vi "Pid.vi"() -> ()   [LabVIEW 2016]
uses:
  <vilib>/Instr/_visa.llb/VISA Configure Serial Port (Instr).vi
panel:
  out "String 2":string
  out "String":string
  out "CM4SpeedPID.ref":i16
  out "CM3SpeedPID.ref":i16
  out "CM2SpeedPID.ref":i16
  out "CM1SpeedPID.ref":i16
  out "ChassisData.ChassisSpeedRef.Omega":i16
  out "ChassisData.ChassisSpeedRef.X":i16
  out "ChassisData.ChassisSpeedRef.Y":i16
  out "GMPitchEncoder.ecd_angle":i16
  out "GMYawEncoder.ecd_angle":i16
  out "GMYawEncoder.ecd_bias":i16
  out "GMYawEncoder.raw_value":i16
  out "GMPitchEncoder.ecd_bias":i16
  out "GMPitchEncoder.raw_value":i16
  out "GMPPositionPID.fdb":i16
  out "GMYPositionPID.fdb":i16
  out "GMPSpeedPID.fdb":i16
  out "GMYSpeedPID.fdb":i16
  out "GMPPositionPID.ref":i16
  out "GMYPositionPID.ref":i16
  out "GMPSpeedPID.ref":i16
  out "GMYSpeedPID.ref":i16
  out "Motor4_Measure.speed_rpm":i16
  out "Motor3_Measure.speed_rpm":i16
  out "Motor2_Measure.speed_rpm":i16
  out "Motor1_Measure.speed_rpm":i16
  out "RC_CtrlData.mouse.y":i16
  out "RC_CtrlData.mouse.x":i16
  out "RC_CtrlData.key.v":i16
  out "RC_CtrlData.rc.s2":i16
  out "RC_CtrlData.rc.s1":i16
  out "RC_CtrlData.rc.ch3":i16
  out "RC_CtrlData.rc.ch1":i16
  out "RC_CtrlData.rc.ch0":i16
  out "RC_CtrlData.rc.ch2":i16
  out "MPU6050_Raw_Data.Gyro_Z":i16
  out "AppParamRealUsed.GyroCaliData.GyroZOffset":i16
  out "AppParamRealUsed.GyroCaliData.GyroYOffset":i16
  out "AppParamRealUsed.GyroCaliData.GyroXOffset":i16
  out "MPU6050_Raw_Data.Gyro_Y":i16
  out "MPU6050_Raw_Data.Gyro_X":i16
  out "MPU6050_Raw_Data.Accel_Z":i16
  out "MPU6050_Raw_Data.Accel_Y":i16
  out "MPU6050_Raw_Data.Accel_X":i16
  out "yaw_angle":i16
  out "roll_angle":i16
  out "pitch_angle":i16
  out "GetChassis_MoveMode":u16
  out "GetGimbal_MoveMode":u16
  out "GetShootState":u16
  out "GetFrictionState":u16
  out "GetAttackMode":u16
  out "GetWorkState":u16
  out "Chassis_MoveMode":string="Nothing"
  out "Gimbal_MoveMode":string="Nothing"
  out "ShootState":string="Nothing"
  out "FrictionState":string="Nothing"
  out "AttackMode":string="Nothing"
  out "WorkState":string="Nothing"
  out "DBUSFrameRate":i16
  out "PitchFrameRate":i16
  out "YawFrameRate":i16
  out "ChassisFrameRate[0]":i16
  out "ChassisFrameRate[1]":i16
  out "ChassisFrameRate[2]":i16
  out "ChassisFrameRate[3]":i16
  out "JudgeFrameRate":i16
  out "IMUFrameRate":i16
  out "MiniPCFrameRate":i16
  out "show num":u32
  out "Init":u8
  out "First?":bool=TRUE
  out "Waveform Chart":dynamicdata(graph)
  in  "ID:":u8=2 format="%x"
  in  "Save":bool
  in  "Show":bool
  in  "File Name:":string="Frame"
  in  "Open":bool
  in  "Baud Rate":u32(ring)=115200 items=["76800"=76800, "100000"=100000, "500000"=500000, "115200"=115200, "9600"=9600]
  in  "Serial port":refnum<visa-resource-name>
  out "Wrong":u64
  out "Right":u64
  in  "unpack":T1 {"Data" format="%x"; "Frame length" format="%x"; "Frame ID" format="%x"}
  in  "Tab Control":enum32{"Gimbal", "Shoot", "Chassis"}(tab)
  in  "Down Picth":bool
  in  "Down Yaw":bool
  out "Down Picth Susess":bool caption="Picth susess"
  out "Down Yaw Susess":bool caption="Picth susess"
  out "Y-S-D 3":u16
  out "Y-S-I 3":u16
  out "Y-S-P 3":u16
  out "Y-P-D 3":u16
  out "Y-P-I 3":u16
  out "Y-P-P 3":u16
  out "P-P-P 3":u16
  out "P-S-D 3":u16
  out "P-S-I 3":u16
  out "P-S-P 3":u16
  out "P-P-D 3":u16
  out "P-P-I 3":u16
  in  "P-P-P 2":u16
  in  "Y-S-D 2":u16
  in  "Y-S-I 2":u16
  in  "Y-S-P 2":u16
  in  "Y-P-D 2":u16
  in  "Y-P-I 2":u16
  in  "Y-P-P 2":u16
  in  "P-S-D 2":u16
  in  "P-S-I 2":u16
  in  "P-S-P 2":u16
  in  "P-P-D 2":u16
  in  "P-P-I 2":u16
  in  "S-P-I":u16
  in  "S-P-D":u16
  in  "S-S-P":u16
  in  "S-S-I":u16
  in  "S-S-D":u16
  in  "S-P-P":u16
  out "S-P-I 4":u16
  out "S-P-D 4":u16
  out "S-S-P 4":u16
  out "S-S-I 4":u16
  out "S-S-D 4":u16
  out "S-P-P 4":u16
  out "T-T-T-S 4":u16
  out "F-W-M-V 4":u16
  out "Down Shoot Susess":bool caption="Picth susess"
  in  "Down Shoot":bool
  in  "T-T-T-S":u16
  in  "F-W-M-V":u16
  in  "R-S-I":u16
  in  "R-S-D":u16
  in  "C-S-P":u16
  in  "C-S-I":u16
  in  "C-S-D":u16
  in  "R-S-P":u16
  out "R-S-I 5":u16
  out "R-S-D 5":u16
  out "C-S-P 5":u16
  out "C-S-I 5":u16
  out "C-S-D 5":u16
  out "R-S-P 5":u16
  out "Down Chassis Susess":bool caption="Picth susess"
  in  "Down Chassis":bool
  in  "Calibrate Gimbal":bool
  out "Calibrate Gimbal Susess":bool caption="Picth susess"
  in  "Calibrate Gyro":bool
  out "Calibrate Gyro Susess":bool caption="Picth susess"
  in  "Calibrate LittleGyro":bool
  out "Calibrate LittleGyro Susess":bool caption="Picth susess"
  # "Position"
  # "Speed"
  # "Position"
  # "Speed"
  # "Pitch"
  # "Yaw"
  # "Pitch"
  # "Yaw"
  # "Position"
  # "Speed"
  # "Position"
  # "Speed"
  # "Turn\nTable"
  # "Turn\nTable"
  # "Turn Table\nTarget speed"
  # "Turn Table\nTarget speed"
  # "Friction Wheel\nMax Value"
  # "Friction Wheel\nMax Value"
  # "Position"
  # "Speed"
  # "Position"
  # "Speed"
  # "Chassis"
  # "Chassis"
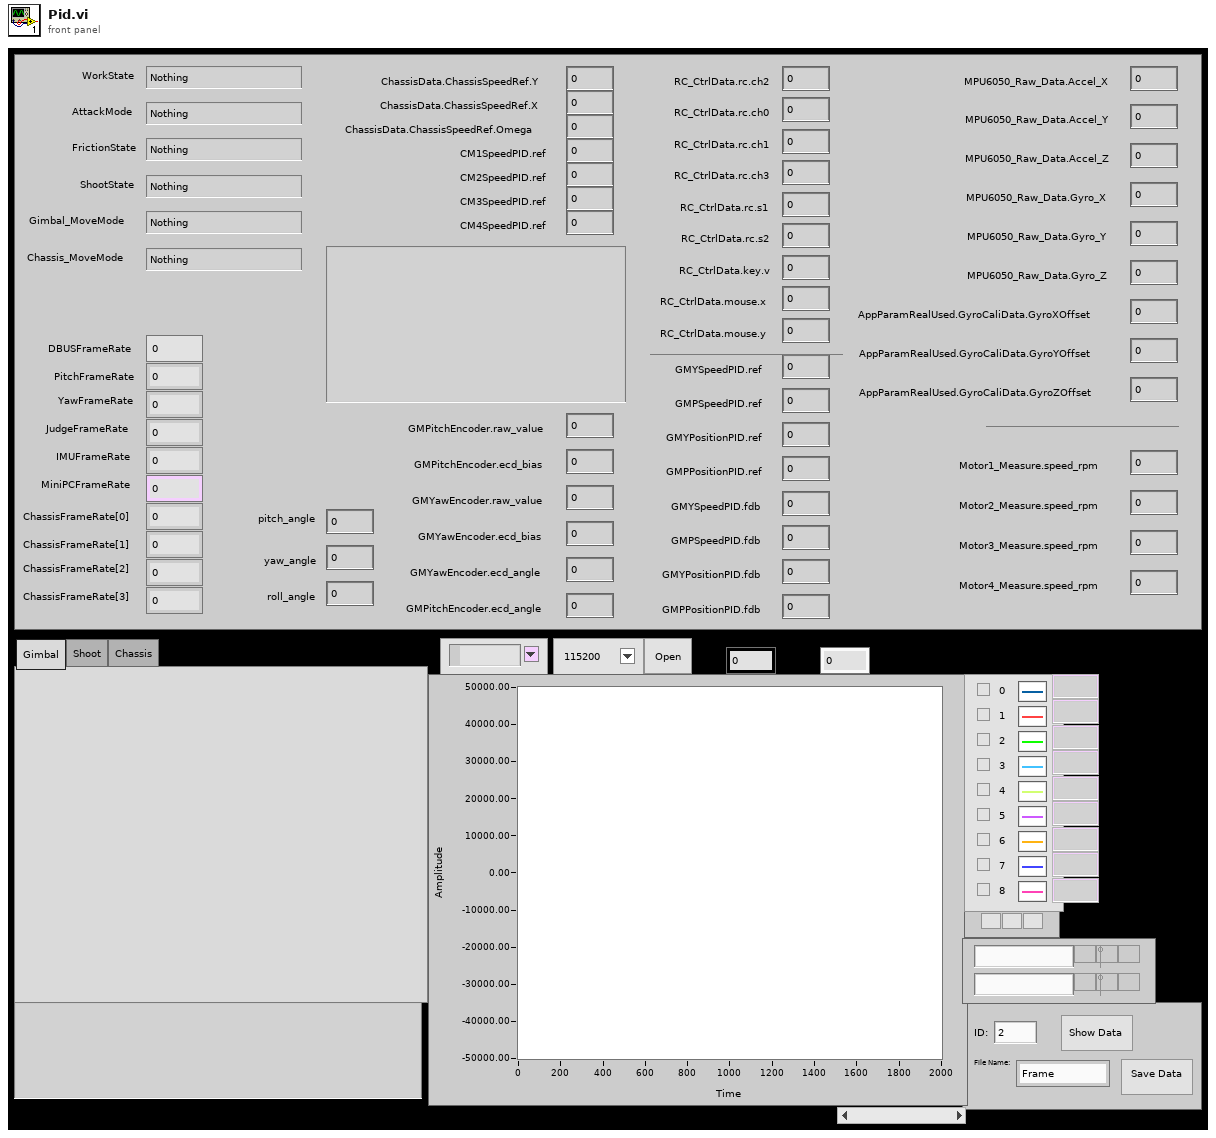
[diagram p1: front panel]
types:
  T1 = cluster{"Status":u8, "Read":u8, "Frame ID":u8, "Frame length":u8, "Data":u8[]}
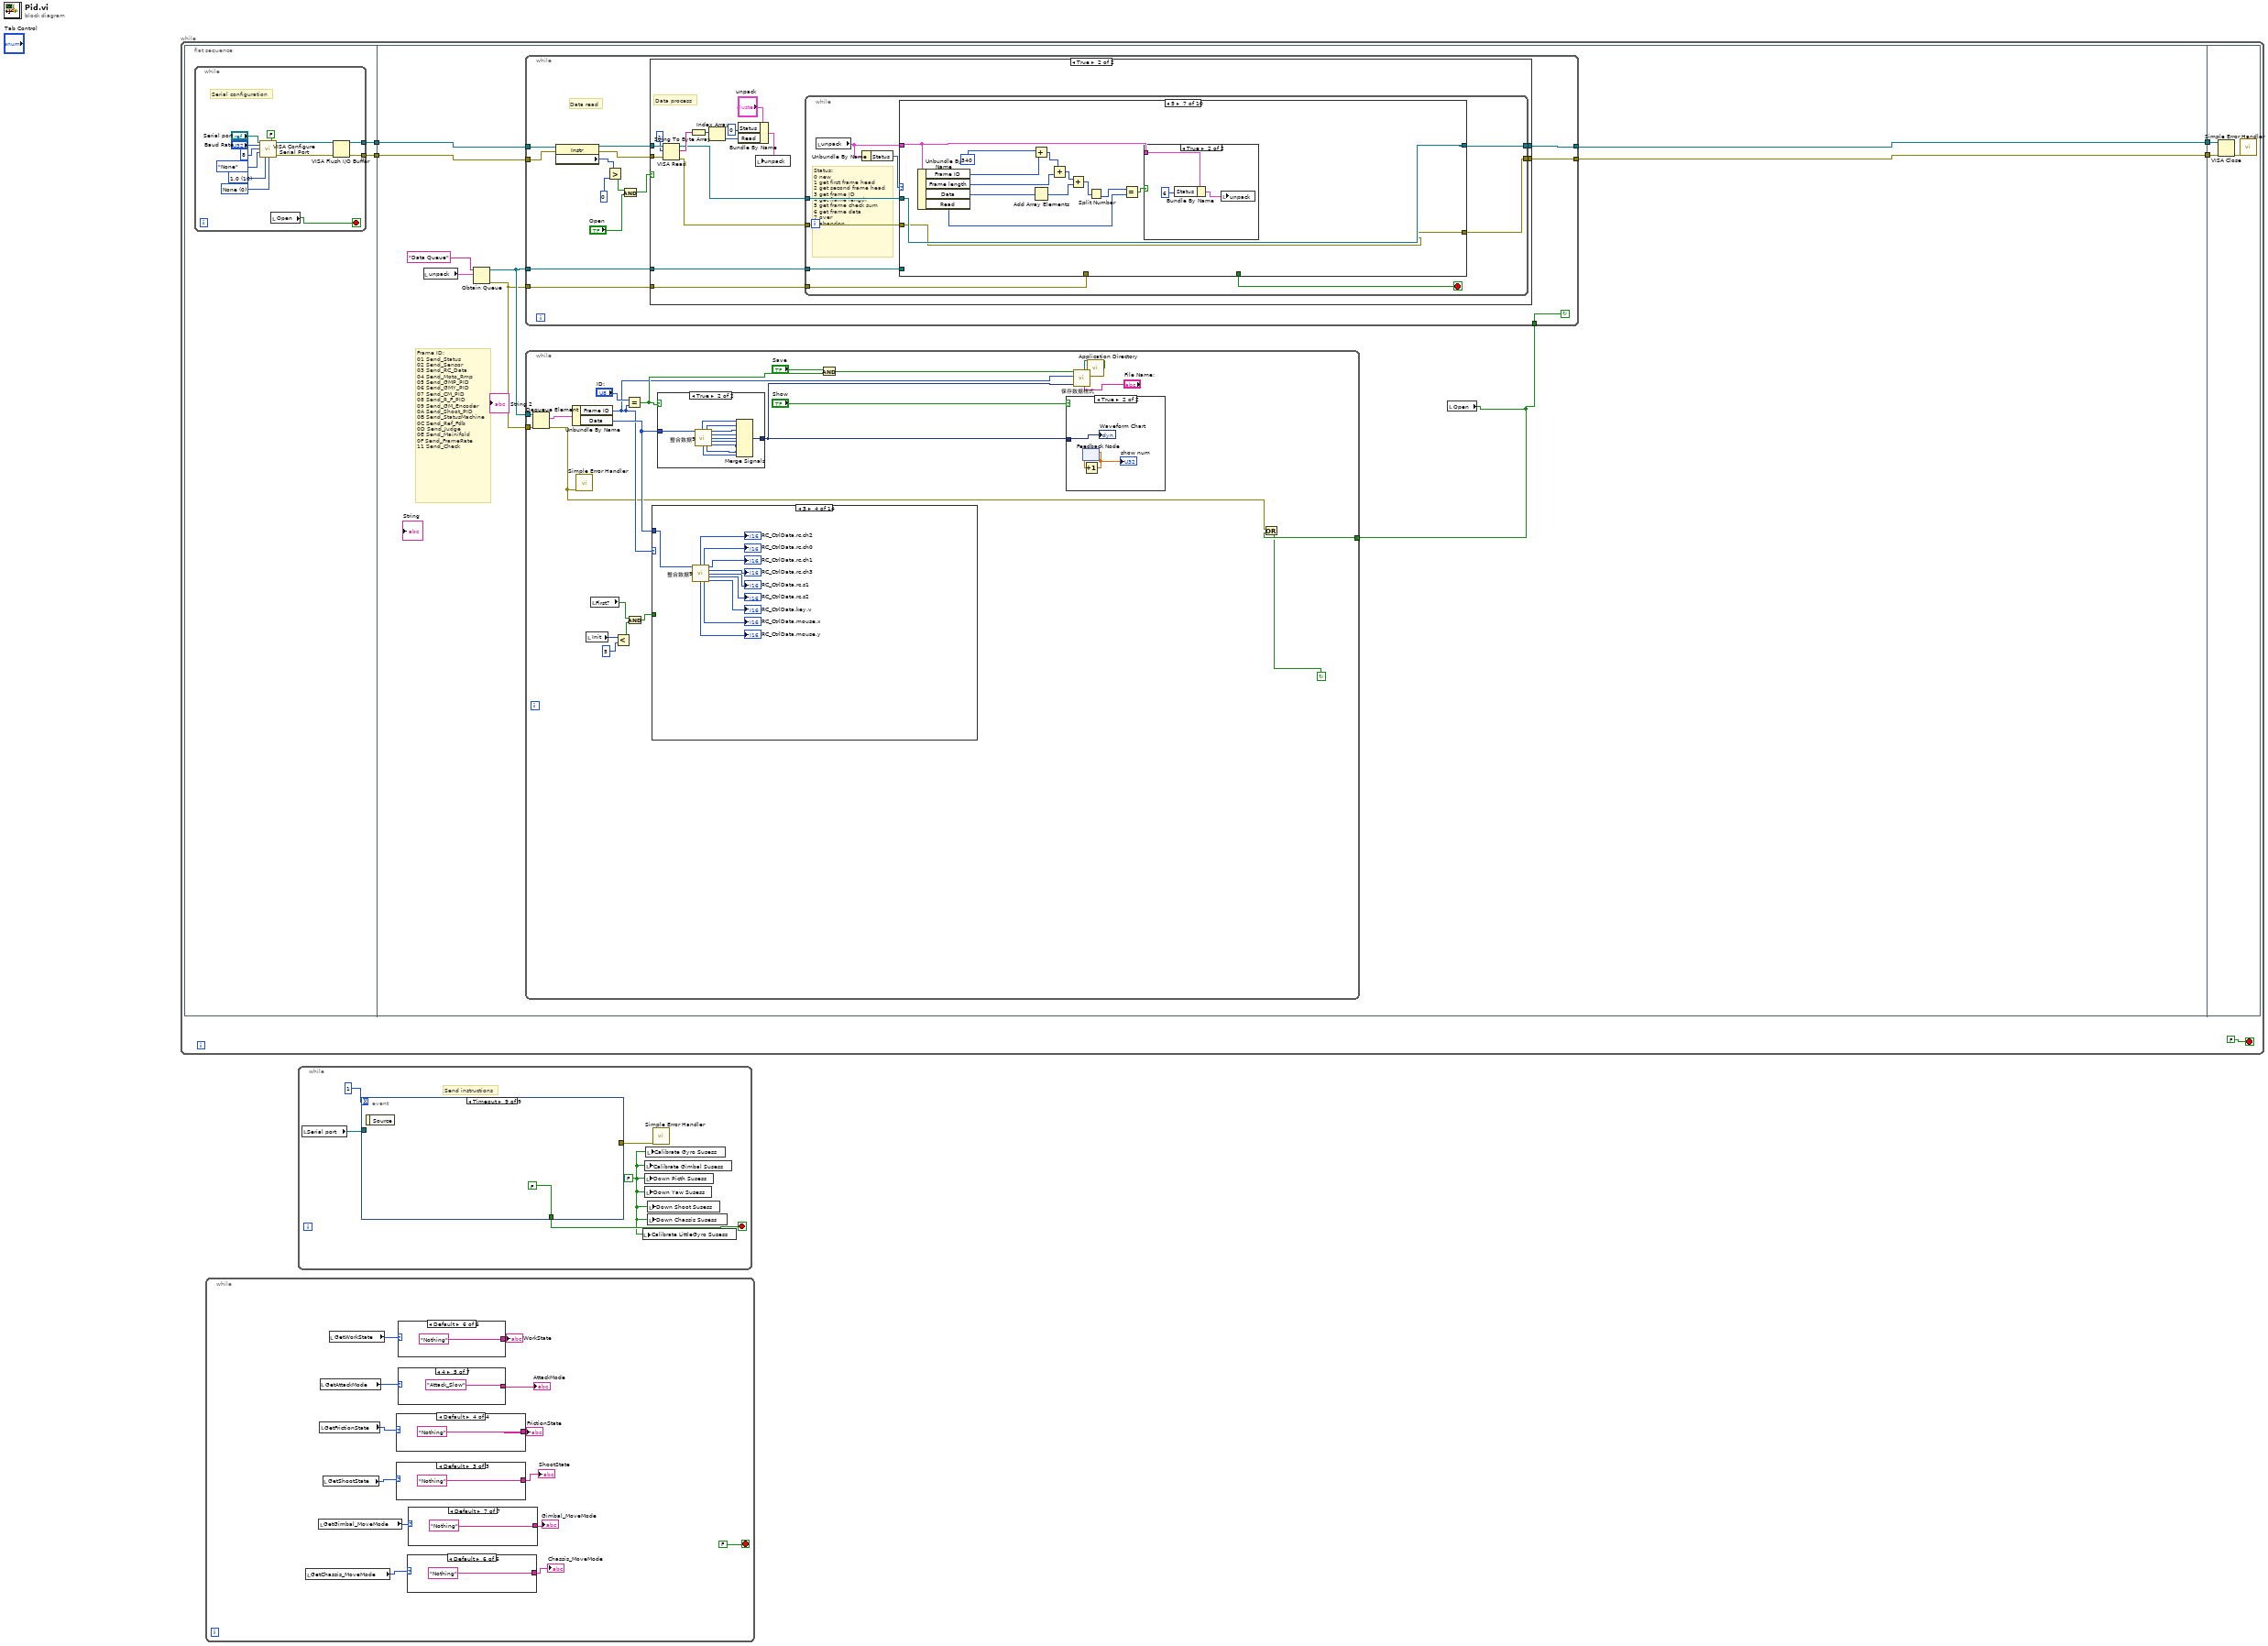
[diagram p0: block diagram]
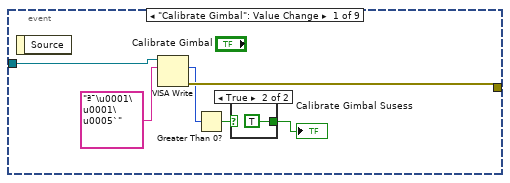
[diagram p2: hidden frame]
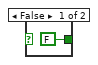
[diagram p3: hidden frame]
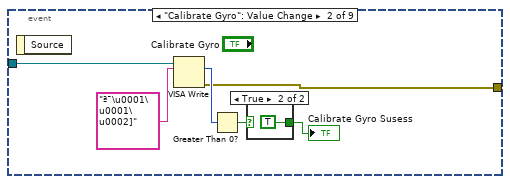
[diagram p4: hidden frame]
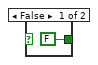
[diagram p5: hidden frame]
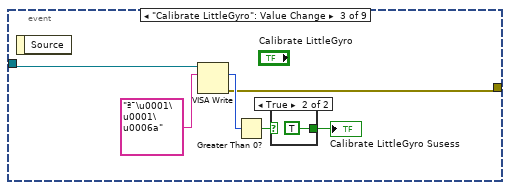
[diagram p6: hidden frame]
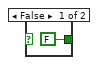
[diagram p7: hidden frame]
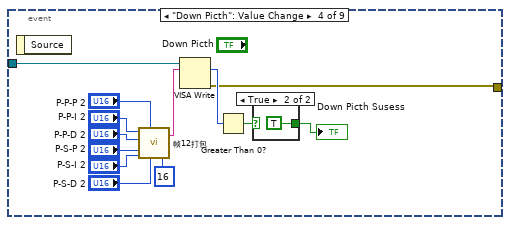
[diagram p8: hidden frame]
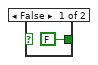
[diagram p9: hidden frame]
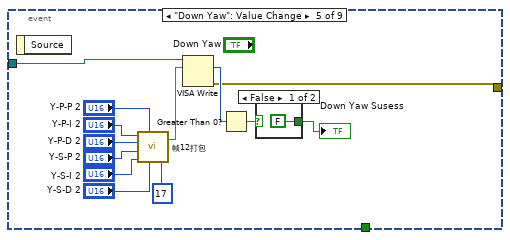
[diagram p10: hidden frame]
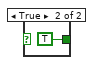
[diagram p11: hidden frame]
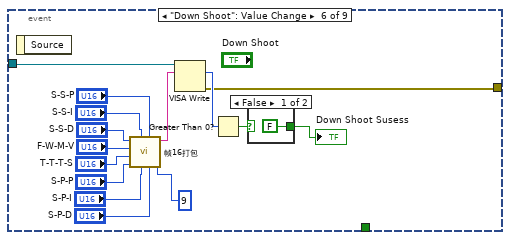
[diagram p12: hidden frame]
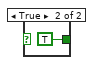
[diagram p13: hidden frame]
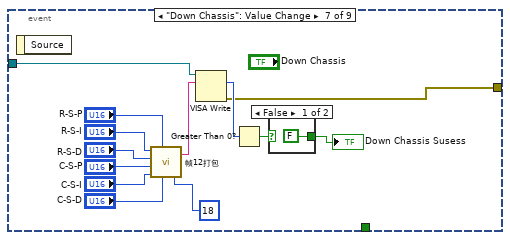
[diagram p14: hidden frame]
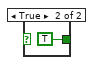
[diagram p15: hidden frame]
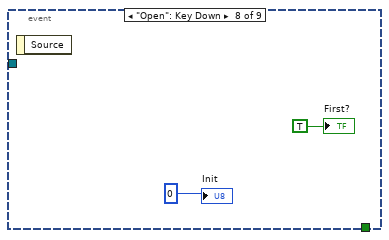
[diagram p16: hidden frame]
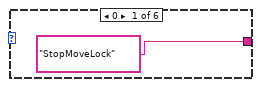
[diagram p17: hidden frame]
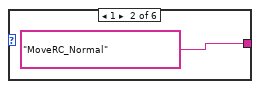
[diagram p18: hidden frame]
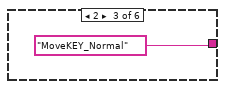
[diagram p19: hidden frame]
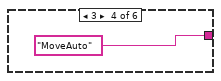
[diagram p20: hidden frame]
diagram:
  n1 = while {
    stop <- FALSE stop-if-true
    n2 = flat-sequence {
      tunnel: [w7] -> w5
      tunnel: [w6] -> w4
      tunnel: w5 -> [w28]
      tunnel: w4 -> [w27]
      tunnel: [w26] -> w3
      tunnel: [w25] -> w2
      tunnel: w3 -> [w368]
      tunnel: w2 -> [w367]
      frame #0 {
        n3 = while {
          tunnel: [w19] -> w7
          tunnel: [w18] -> w6
          stop <- w8 stop-if-true
          w11 = u16 0 items=["None", "XON/XOFF", "RTS/CTS", "XON/XOFF & RTS/CTS", "DTR/DSR", "XON/XOFF & DTR/DSR"] ("flow control (0:none)")
          w12 = u16 10 items=["1.0"=10, "1.5"=15, "2.0"=20] ("stop bits (10: 1 bit)")
          # "Serial configuration"
          n4 = call-poly "VISA Configure Serial Port"("VISA resource name"="Serial port", "Enable Termination\nChar (T)"=FALSE ("Enable Termination\nChar (T)"), "baud rate (9600)"="Baud Rate", "data bits (8)"=u16 8, "parity (0:none)"=enum16{"None", "Odd", "Even", "Mark", "Space"}."None", "stop bits (10: 1 bit)"=w12, "flow control (0:none)"=w11) -> ("VISA resource name out"=w9:refnum<visa-resource-name>, "error out"=w10:errorcluster)  [unwired: 7 in]
          n5 = local read "Open"() -> (w8:bool)
          n6 = VISA Flush I/O Buffer(VISA resource name=w9, error in (no error)=w10) -> (VISA resource name out=w19:refnum<visa-resource-name>, error out=w18:errorcluster)  [unwired: 1 in]
        }
      }
      frame #1 {
        # "Frame ID:\n01 Send_Status\n02 Send_Sensor\n03 Send_RC_Data\n04 Send_Moto_Rmp\n05 Send_GMP_PID\n06 Send_GMY_PID\n07 Send_CM_PID\n08 Send_R_F_PID\n09 Send_GM_Encoder\n0A Send_Shoot_PID\n0B Send_StatusMachine\n0C Send_Ref_Fdb\n0D Send_Judge\n0E Send_Mainifold\n0F Send_FrameRate\n11 Send_Check"
        n7 = local read "unpack"() -> (w24:T1)
        n8 = Obtain Queue(name (unnamed)="Data Queue", element data type=w24) -> (queue out=w22:refnum<queue>, error out=w21:errorcluster)  [unwired: 3 in, 1 out]
        n9 = local read "Open"() -> (w20:bool)
        n10 = while {
          tunnel: w28 -> [w231]
          tunnel: w27 -> [w230]
          tunnel: [w233] -> w26
          tunnel: [w232] -> w25
          tunnel: w22 -> [w222]
          tunnel: w21 -> [w221]
          tunnel: w20 -> [w220]
          stop <- w220 continue-if-true
          # "Data read"
          n11 = property class="Instr"(reference=w231, error in=w230) -> (reference out=w228:refnum<visa-resource-name>, error out=w229:errorcluster, "Serial Settings:Number of Bytes at Serial Port"=w227:u32)
          n12 = Greater?(x=w227, y=0) -> (0:w225:bool)
          n13 = And(x=w225, y="Open") -> (x .and. y?=w224:bool)
          n14 = case shown="True" w224 {
            tunnel: [w234 w239] -> w232
            tunnel: [w235 w240] -> w233
            tunnel: w228 -> [w235 w250]
            tunnel: w229 -> [w234 w249]
            tunnel: w222 -> [_ w237]
            tunnel: w221 -> [_ w236]
            frame False {
            }
            frame True {
              # "Data process"
              n15 = VISA Read(VISA resource name=w250, byte count=u8 1, error in (no error)=w249) -> (VISA resource name out=w242:refnum<visa-resource-name>, read buffer=w244:string, error out=w241:errorcluster)  [unwired: 1 out]
              n16 = String To Byte Array(string=w244) -> (unsigned byte array=w247:u8[])
              n17 = Index Array(array=w247) -> (element=w246:u8)  [unwired: 1 in]
              n18 = Bundle By Name(cluster="unpack", "Status"=u8 0, "Read"=w246) -> (w238:T1)
              n19 = local write "unpack"(w238) -> ()
              n20 = while {
                tunnel: w242 -> [w257]
                tunnel: w241 -> [w256]
                tunnel: [w255] -> w240
                tunnel: [w254] -> w239
                tunnel: w237 -> [w252]
                tunnel: w236 -> [w251]
                stop <- w258 stop-if-true
                # "Status:\n0 new\n1 get first frame head\n2 get second frame head\n3 get frame ID\n4 get frame length\n5 get frame check sum\n6 get frame data\n7 over\n8 abandon"
                n21 = local read "unpack"() -> (w253:T1)
                n22 = Unbundle By Name(w253) -> ("Status"=w259:u8)
                n23 = case shown="5" w259 {
                  tunnel: w253 -> [_ w264 w278 w298 w307 w324 w336 w355 _ _]
                  tunnel: [_ _ _ _ _ _ _ _ TRUE TRUE] -> w258
                  tunnel: w257 -> [w261 w263 w277 w296 w306 w322 w328 w352 w357 w362]
                  tunnel: w256 -> [w260 w262 w276 w295 w305 w321 w327 w350 w356 w361]
                  tunnel: [w261 w263 w275 w294 w304 w320 w328 w352 w357 w362] -> w255
                  tunnel: [w260 w262 w274 w293 w303 w319 w327 w350 w356 w361] -> w254
                  tunnel: w252 -> [_ _ _ _ _ _ _ w348 _ _]
                  tunnel: w251 -> [_ _ _ _ _ _ _ w347 _ _]
                  frame Default {
                  }
                  frame 0 {
                    n24 = Unbundle By Name(w264) -> ("Read"=w267:u8)
                    n25 = Equal?(x=u8 170, y=w267) -> (x = y?=w265:bool)
                    n26 = case shown="False" w265 {
                      tunnel: w264 -> [w269 w272]
                      frame False {
                        n27 = Bundle By Name(cluster=w269, "Status"=u8 8) -> (w268:T1)
                        n28 = local write "unpack"(w268) -> ()
                      }
                      frame True {
                        n29 = Bundle By Name(cluster=w272, "Status"=u8 1) -> (w271:T1)
                        n30 = local write "unpack"(w271) -> ()
                      }
                    }
                  }
                  frame 1 {
                    n31 = VISA Read(VISA resource name=w277, byte count=u8 1, error in (no error)=w276) -> (VISA resource name out=w275:refnum<visa-resource-name>, read buffer=w283:string, error out=w274:errorcluster)  [unwired: 1 out]
                    n32 = String To Byte Array(string=w283) -> (unsigned byte array=w282:u8[])
                    n33 = Index Array(array=w282) -> (element=w281:u8)  [unwired: 1 in]
                    n34 = Equal?(x=u8 170, y=w281) -> (x = y?=w279:bool)
                    n35 = case shown="False" w279 {
                      tunnel: w278 -> [w287 w290]
                      frame False {
                        n36 = Bundle By Name(cluster=w287, "Status"=u8 8) -> (w285:T1)
                        n37 = local write "unpack"(w285) -> ()
                      }
                      frame True {
                        n38 = Bundle By Name(cluster=w290, "Status"=u8 2) -> (w288:T1)
                        n39 = local write "unpack"(w288) -> ()
                      }
                    }
                  }
                  frame 2 {
                    n40 = VISA Read(VISA resource name=w296, byte count=u8 1, error in (no error)=w295) -> (VISA resource name out=w294:refnum<visa-resource-name>, read buffer=w300:string, error out=w293:errorcluster)  [unwired: 1 out]
                    n41 = String To Byte Array(string=w300) -> (unsigned byte array=w301:u8[])
                    n42 = Index Array(array=w301) -> (element=w291:u8)  [unwired: 1 in]
                    n43 = Bundle By Name(cluster=w298, "Status"=u8 3, "Frame ID"=w291) -> (w292:T1)
                    n44 = local write "unpack"(w292) -> ()
                  }
                  frame 3 {
                    n45 = VISA Read(VISA resource name=w306, byte count=u8 1, error in (no error)=w305) -> (VISA resource name out=w304:refnum<visa-resource-name>, read buffer=w309:string, error out=w303:errorcluster)  [unwired: 1 out]
                    n46 = String To Byte Array(string=w309) -> (unsigned byte array=w308:u8[])
                    n47 = Index Array(array=w308) -> (element=w312:u8)  [unwired: 1 in]
                    n48 = Bundle By Name(cluster=w307, "Status"=u8 4, "Frame length"=w312) -> (w302:T1)
                    n49 = local write "unpack"(w302) -> ()
                  }
                  frame 4 {
                    n50 = Unbundle By Name(w324) -> ("Frame length"=w313:u8)
                    n51 = Increment(x=w313) -> (x+1=w325:u8)
                    n52 = VISA Read(VISA resource name=w322, byte count=w325, error in (no error)=w321) -> (VISA resource name out=w320:refnum<visa-resource-name>, read buffer=w315:string, error out=w319:errorcluster)  [unwired: 1 out]
                    n53 = String To Byte Array(string=w315) -> (unsigned byte array=w323:u8[])
                    n54 = Index Array(array=w323, index=w313) -> (element=w316:u8)
                    n55 = Array Subset(array=w323, index=u8 0, length=w313) -> (w314:u8[])
                    n56 = Bundle By Name(cluster=w324, "Status"=u8 5, "Read"=w316, "Data"=w314) -> (w318:T1)
                    n57 = local write "unpack"(w318) -> ()
                  }
                  frame 5 {
                    n58 = Unbundle By Name(w336) -> ("Frame ID"=w334:u8, "Frame length"=w332:u8, "Data"=w340:u8[], "Read"=w338:u8)
                    n59 = Add(x=u16 340, y=w334) -> (x+y=w333:u16)
                    n60 = Add Array Elements(numeric array=w340) -> (sum=w330:u8)
                    n61 = Add(x=w333, y=w332) -> (x+y=w331:u16)
                    n62 = Add(x=w331, y=w330) -> (x+y=w329:u16)
                    n63 = Split Number(x=w329) -> (lo(x)=w339:u8)  [unwired: 1 out]
                    n64 = Equal?(x=w339, y=w338) -> (x = y?=w337:bool)
                    n65 = case shown="True" w337 {
                      tunnel: w336 -> [w342 w346]
                      frame False {
                        n66 = Bundle By Name(cluster=w342, "Status"=u8 8) -> (w341:T1)
                        n67 = local write "unpack"(w341) -> ()
                      }
                      frame True {
                        n68 = Bundle By Name(cluster=w346, "Status"=u8 6) -> (w344:T1)
                        n69 = local write "unpack"(w344) -> ()
                      }
                    }
                  }
                  frame 6 {
                    n70 = Bundle By Name(cluster=w355, "Status"=u8 7) -> (w353:T1)
                    n71 = local write "unpack"(w353) -> ()
                    n72 = local read "unpack"() -> (w351:T1)
                    n73 = Enqueue Element(queue=w348, element=w351, error in (no error)=w347) -> (error out=w349:errorcluster)  [unwired: 1 in, 2 out]
                    n74 = call <vilib>:"Simple Error Handler.vi"("error in (no error)"=w349) -> ()  [unwired: 2 in, 7 out]
                  }
                  frame 7 {
                    n75 = feedback #1() -> (w359:dbl)  [unwired: 1 in]
                    n76 = Increment(x=w359) -> (x+1=w358:dbl)
                    "Right" <- w358
                    n77 = feedback-in #1(w358) -> ()
                  }
                  frame 8 {
                    n78 = feedback #2() -> (w364:dbl)  [unwired: 1 in]
                    n79 = Increment(x=w364) -> (x+1=w363:dbl)
                    "Wrong" <- w363
                    n80 = feedback-in #2(w363) -> ()
                  }
                }
              }
            }
          }
        }
        n81 = while {
          tunnel: w22 -> [w41]
          tunnel: w21 -> [w40]
          tunnel: w20 -> [w30]
          stop <- w29 continue-if-true
          n82 = Dequeue Element(queue=w41, error in (no error)=w40) -> (element=w42:T1, error out=w31:errorcluster)  [unwired: 1 in, 2 out]
          n83 = Unbundle By Name(w42) -> ("Frame ID"=w32:u8, "Data"=w33:u8[])
          n84 = call <vilib>:"Simple Error Handler.vi"("error in (no error)"=w31) -> ()  [unwired: 2 in, 7 out]
          n85 = local read "Init"() -> (w39:u8)
          n86 = local read "First?"() -> (w37:bool)
          n87 = Less?(x=w39, y=u8 5) -> (x < y?=w36:bool)
          n88 = Equal?(x="ID:", y=w32) -> (x = y?=w47:bool)
          n89 = And(x=w37, y=w36) -> (x .and. y?=w35:bool)
          n90 = case shown="3" w32 {
            tunnel: w33 -> [_ w60 w70 w80 w85 w93 w110 w126 w148 w158 w172 w189 w197 w208]
            tunnel: w35 -> [_ _ _ _ _ w92 w109 w119 _ _ w171 _ _ _]
            frame Default {
            }
            frame 1 {
              w59 = 100
              n91 = call "整合数据6.vi"("Data in"=w60) -> ("P1"=w58:u16, "I1"=w57:u16, "D1"=w56:u16)  [unwired: 4 in, 3 out]
              n92 = Divide(x=w58, y=w59) -> (x/y=→"pitch_angle":dbl)
              n93 = Divide(x=w57, y=w59) -> (x/y=→"roll_angle":dbl)
              n94 = Divide(x=w56, y=w59) -> (x/y=→"yaw_angle":dbl)
            }
            frame 2 {
              n95 = call "整合数据9.vi"("Data in"=w70) -> ("P1"=→"MPU6050_Raw_Data.Accel_X":i16, "I1"=→"MPU6050_Raw_Data.Accel_Y":i16, "D1"=→"MPU6050_Raw_Data.Accel_Z":i16, "P2"=→"MPU6050_Raw_Data.Gyro_X":i16, "I2"=→"MPU6050_Raw_Data.Gyro_Y":i16, "D2"=→"MPU6050_Raw_Data.Gyro_Z":i16, "D3"=→"AppParamRealUsed.GyroCaliData.GyroZOffset":i16, "I3"=→"AppParamRealUsed.GyroCaliData.GyroYOffset":i16, "P3"=→"AppParamRealUsed.GyroCaliData.GyroXOffset":i16)  [unwired: 6 in]
            }
            frame 3 {
              n96 = call "整合数据9.vi"("Data in"=w80) -> ("P1"=→"RC_CtrlData.rc.ch2":i16, "I1"=→"RC_CtrlData.rc.ch0":i16, "D1"=→"RC_CtrlData.rc.ch1":i16, "P2"=→"RC_CtrlData.rc.ch3":i16, "I2"=→"RC_CtrlData.rc.s1":i16, "D2"=→"RC_CtrlData.rc.s2":i16, "D3"=→"RC_CtrlData.mouse.y":i16, "I3"=→"RC_CtrlData.mouse.x":i16, "P3"=→"RC_CtrlData.key.v":i16)  [unwired: 6 in]
            }
            frame 4 {
              n97 = call "整合数据6.vi"("Data in"=w85) -> ("P1"=→"Motor1_Measure.speed_rpm":u16, "I1"=→"Motor2_Measure.speed_rpm":u16, "D1"=→"Motor3_Measure.speed_rpm":u16, "P2"=→"Motor4_Measure.speed_rpm":u16)  [unwired: 4 in, 2 out]
            }
            frame 5 {
              n98 = call "整合数据6.vi"("Data in"=w93) -> ("P1"=w91:u16, "I1"=w90:u16, "D1"=w89:u16, "D2"=w86:u16, "P2"=w88:u16, "I2"=w87:u16)  [unwired: 4 in]
              "P-P-I 3" <- w90
              "P-S-I 3" <- w87
              "P-P-P 3" <- w91
              "P-S-D 3" <- w86
              "P-P-D 3" <- w89
              "P-S-P 3" <- w88
              n99 = case shown="False" w92 {
                tunnel: w91 -> [_ w100]
                tunnel: w90 -> [_ w99]
                tunnel: w89 -> [_ w98]
                tunnel: w88 -> [_ w97]
                tunnel: w87 -> [_ w96]
                tunnel: w86 -> [_ w95]
                frame False {
                  n100 = local write "First?"(FALSE) -> ()
                }
                frame True {
                  n101 = local read "Init"() -> (w101:u8)
                  n102 = local write "P-P-P 2"(w100) -> ()
                  n103 = local write "P-P-I 2"(w99) -> ()
                  n104 = local write "P-P-D 2"(w98) -> ()
                  n105 = local write "P-S-P 2"(w97) -> ()
                  n106 = local write "P-S-I 2"(w96) -> ()
                  n107 = local write "P-S-D 2"(w95) -> ()
                  n108 = Increment(x=w101) -> (x+1=w102:u8)
                  n109 = local write "Init"(w102) -> ()
                }
              }
            }
            frame 6 {
              n110 = call "整合数据6.vi"("Data in"=w110) -> ("P1"=w108:u16, "I1"=w107:u16, "D1"=w106:u16, "D2"=w103:u16, "P2"=w105:u16, "I2"=w104:u16)  [unwired: 4 in]
              "Y-P-P 3" <- w108
              "Y-P-I 3" <- w107
              "Y-P-D 3" <- w106
              "Y-S-I 3" <- w104
              "Y-S-D 3" <- w103
              "Y-S-P 3" <- w105
              n111 = case shown="True" w109 {
                tunnel: w108 -> [_ w116]
                tunnel: w107 -> [_ w115]
                tunnel: w106 -> [_ w114]
                tunnel: w105 -> [_ w113]
                tunnel: w104 -> [_ w112]
                tunnel: w103 -> [_ w111]
                frame False {
                }
                frame True {
                  n112 = local read "Init"() -> (w118:u8)
                  n113 = local write "Y-P-P 2"(w116) -> ()
                  n114 = local write "Y-P-I 2"(w115) -> ()
                  n115 = local write "Y-P-D 2"(w114) -> ()
                  n116 = local write "Y-S-P 2"(w113) -> ()
                  n117 = local write "Y-S-I 2"(w112) -> ()
                  n118 = local write "Y-S-D 2"(w111) -> ()
                  n119 = Increment(x=w118) -> (x+1=w117:u8)
                  n120 = local write "Init"(w117) -> ()
                }
              }
            }
            frame 7 {
              n121 = call "整合数据6.vi"("Data in"=w126) -> ("P1"=w125:u16, "I1"=w124:u16, "D1"=w123:u16, "D2"=w120:u16, "P2"=w122:u16, "I2"=w121:u16)  [unwired: 4 in]
              "R-S-I 5" <- w124
              "R-S-D 5" <- w123
              "C-S-P 5" <- w122
              "C-S-I 5" <- w121
              "C-S-D 5" <- w120
              "R-S-P 5" <- w125
              n122 = case shown="True" w119 {
                tunnel: w125 -> [_ w132]
                tunnel: w124 -> [_ w131]
                tunnel: w123 -> [_ w130]
                tunnel: w122 -> [_ w129]
                tunnel: w121 -> [_ w128]
                tunnel: w120 -> [_ w127]
                frame False {
                }
                frame True {
                  n123 = local read "Init"() -> (w133:u8)
                  n124 = Increment(x=w133) -> (x+1=w134:u8)
                  n125 = local write "R-S-P"(w132) -> ()
                  n126 = local write "R-S-I"(w131) -> ()
                  n127 = local write "R-S-D"(w130) -> ()
                  n128 = local write "C-S-P"(w129) -> ()
                  n129 = local write "C-S-I"(w128) -> ()
                  n130 = local write "C-S-D"(w127) -> ()
                  n131 = local write "Init"(w134) -> ()
                }
              }
            }
            frame 8 {
              w143 = 100
              n132 = call "整合数据9.vi"("Data in"=w148) -> ("P1"=→"GMYSpeedPID.ref":i16, "I1"=→"GMPSpeedPID.ref":i16, "D1"=w142:i16, "P2"=w141:i16, "I2"=→"GMYSpeedPID.fdb":i16, "D2"=→"GMPSpeedPID.fdb":i16, "I3"=w139:i16, "P3"=w140:i16)  [unwired: 6 in, 1 out]
              n133 = Divide(x=w140, y=w143) -> (x/y=→"GMYPositionPID.fdb":dbl)
              n134 = Divide(x=w139, y=w143) -> (x/y=→"GMPPositionPID.fdb":dbl)
              n135 = Divide(x=w142, y=w143) -> (x/y=→"GMYPositionPID.ref":dbl)
              n136 = Divide(x=w141, y=w143) -> (x/y=→"GMPPositionPID.ref":dbl)
            }
            frame 9 {
              w153 = 100
              n137 = call "整合数据9.vi"("Data in"=w158) -> ("P1"=→"GMPitchEncoder.raw_value":i16, "I1"=→"GMPitchEncoder.ecd_bias":i16, "P2"=→"GMYawEncoder.raw_value":i16, "I2"=→"GMYawEncoder.ecd_bias":i16, "I3"=w151:i16, "P3"=w152:i16)  [unwired: 6 in, 3 out]
              n138 = Divide(x=w152, y=w153) -> (x/y=→"GMYawEncoder.ecd_angle":dbl)
              n139 = Divide(x=w151, y=w153) -> (x/y=→"GMPitchEncoder.ecd_angle":dbl)
            }
            frame 10 {
              w165 = 100
              n140 = call "整合数据9.vi"("Data in"=w172) -> ("P1"=w164:i16, "I1"=w163:i16, "D1"=w170:i16, "P2"=w169:i16, "I2"=w168:i16, "D2"=w167:i16, "I3"=w166:i16, "P3"=w162:i16)  [unwired: 6 in, 1 out]
              "S-P-P 4" <- w167
              "S-S-D 4" <- w170
              "S-P-D 4" <- w166
              "T-T-T-S 4" <- w168
              "F-W-M-V 4" <- w169
              n141 = Divide(x=w164, y=w165) -> (x/y=w159:dbl)
              "S-S-P 4" <- w159
              n142 = Divide(x=w163, y=w165) -> (x/y=w160:dbl)
              "S-S-I 4" <- w160
              n143 = Divide(x=w162, y=w165) -> (x/y=w161:dbl)
              "S-P-I 4" <- w161
              n144 = case shown="True" w171 {
                tunnel: w159 -> [_ w182]
                tunnel: w160 -> [_ w181]
                tunnel: w170 -> [_ w180]
                tunnel: w169 -> [_ w179]
                tunnel: w168 -> [_ w178]
                tunnel: w167 -> [_ w177]
                tunnel: w161 -> [_ w176]
                tunnel: w166 -> [_ w175]
                frame False {
                }
                frame True {
                  n145 = local read "Init"() -> (w173:u8)
                  n146 = Increment(x=w173) -> (x+1=w174:u8)
                  n147 = local write "Init"(w174) -> ()
                  n148 = local write "S-S-P"(w182) -> ()
                  n149 = local write "S-S-I"(w181) -> ()
                  n150 = local write "S-S-D"(w180) -> ()
                  n151 = local write "F-W-M-V"(w179) -> ()
                  n152 = local write "T-T-T-S"(w178) -> ()
                  n153 = local write "S-P-P"(w177) -> ()
                  n154 = local write "S-P-I"(w176) -> ()
                  n155 = local write "S-P-D"(w175) -> ()
                }
              }
            }
            frame 11 {
              n156 = call "整合数据6.vi"("Data in"=w189) -> ("P1"=→"GetWorkState":u16, "I1"=→"GetAttackMode":u16, "D1"=→"GetFrictionState":u16, "D2"=→"GetChassis_MoveMode":u16, "P2"=→"GetShootState":u16, "I2"=→"GetGimbal_MoveMode":u16)  [unwired: 4 in]
            }
            frame 12 {
              n157 = call "整合数据9.vi"("Data in"=w197) -> ("D1"=→"ChassisData.ChassisSpeedRef.Y":i16, "P2"=→"ChassisData.ChassisSpeedRef.X":i16, "I2"=→"ChassisData.ChassisSpeedRef.Omega":i16, "D2"=→"CM1SpeedPID.ref":i16, "D3"=→"CM4SpeedPID.ref":i16, "I3"=→"CM3SpeedPID.ref":i16, "P3"=→"CM2SpeedPID.ref":i16)  [unwired: 6 in, 2 out]
            }
            frame 15 {
              n158 = call "整合数据10.vi"("Data in"=w208) -> ("P1"=→"DBUSFrameRate":i16, "I1"=→"PitchFrameRate":i16, "D1"=→"YawFrameRate":i16, "P2"=→"ChassisFrameRate[0]":i16, "I2"=→"ChassisFrameRate[1]":i16, "D2"=→"ChassisFrameRate[2]":i16, "10"=→"MiniPCFrameRate":i16, "D3"=→"IMUFrameRate":i16, "I3"=→"JudgeFrameRate":i16, "P3"=→"ChassisFrameRate[3]":i16)  [unwired: 5 in]
            }
          }
          n159 = case shown="True" w47 {
            tunnel: w33 -> [_ w219]
            tunnel: [_ w218] -> w45
            frame False {
            }
            frame True {
              n160 = call "整合数据9.vi"("Data in"=w219) -> ("P1"=w217:i16, "I1"=w216:i16, "D1"=w215:i16, "P2"=w214:i16, "I2"=w213:i16, "D2"=w212:i16, "D3"=w209:i16, "I3"=w210:i16, "P3"=w211:i16)  [unwired: 6 in]
              n161 = Merge Signals(w217, w216, w215, w214, w213, w212, w211, w210, w209) -> (w218:dynamicdata)
            }
          }
          n162 = And(x="Save", y=w47) -> (x .and. y?=w48:bool)
          n163 = case shown="True" "Show" {
            tunnel: w45 -> [_ w52]
            frame False {
            }
            frame True {
              n164 = feedback #3() -> (w51:dbl)  [unwired: 1 in]
              n165 = Increment(x=w51) -> (x+1=w50:dbl)
              "show num" <- w50
              n166 = feedback-in #3(w50) -> ()
              "Waveform Chart" <- w52
            }
          }
          n167 = call <vilib>:"Application Directory.vi"() -> ("Application Directory"=w44:path)
          n168 = call "保存数据格式.vi"("Name"="File Name:", "Path"=w44, "数据"=w45, "ID"=w32, "是否保存"=w48) -> ()  [unwired: 7 in]
          n169 = Or(x=w31, y=w30) -> (x .or. y?=w29:bool)
        }
      }
      frame #2 {
        n170 = VISA Close(VISA resource name=w368, error in (no error)=w367) -> (error out=w366:errorcluster)
        n171 = call <vilib>:"Simple Error Handler.vi"("error in (no error)"=w366) -> ()  [unwired: 2 in, 7 out]
      }
    }
  }
  n172 = while {
    stop <- FALSE stop-if-true
    n173 = local read "GetChassis_MoveMode"() -> (w371:u16)
    n174 = local read "GetGimbal_MoveMode"() -> (w373:u16)
    n175 = local read "GetFrictionState"() -> (w376:u16)
    n176 = local read "GetAttackMode"() -> (w378:u16)
    n177 = local read "GetShootState"() -> (w374:u16)
    n178 = local read "GetWorkState"() -> (w381:u16)
    n179 = case shown="Default" w376 {
      tunnel: ["FRICTION_WHEEL_OFF" "FRICTION_WHEEL_START_TURNNING" "FRICTION_WHEEL_ON" "Nothing"] -> w377
      frame 0 {
      }
      frame 1 {
      }
      frame 2 {
      }
      frame Default {
      }
    }
    "FrictionState" <- w377
    n180 = case shown="Default" w374 {
      tunnel: ["NOSHOOTING" "SHOOTING" "Nothing"] -> w375
      frame 0 {
      }
      frame 1 {
      }
      frame Default {
      }
    }
    "ShootState" <- w375
    n181 = case shown="Default" w381 {
      tunnel: ["PREPARE_STATE" "NORMAL_AUTO_STATE" "NORMAL_RC_STATE" "STOP_STATE" "CALI_STATE" "Nothing"] -> w380
      frame 0 {
      }
      frame 1 {
      }
      frame 2 {
      }
      frame 3 {
      }
      frame 4 {
      }
      frame Default {
      }
    }
    "WorkState" <- w380
    n182 = case shown="4" w378 {
      tunnel: ["Attack_Normal" "Attack_HalfAuto" "Attack_Dragon" "Attack_CatWalk" "Attack_Slow" "Attack_45Degree" "Nothing"] -> w379
      frame 0 {
      }
      frame 1 {
      }
      frame 2 {
      }
      frame 3 {
      }
      frame 4 {
      }
      frame 5 {
      }
      frame Default {
      }
    }
    "AttackMode" <- w379
    n183 = case shown="Default" w371 {
      tunnel: ["StopMoveLock" "MoveRC_Normal" "MoveKEY_Normal" "MoveAuto" "MoveFullAuto" "Nothing"] -> w370
      frame 0 {
      }
      frame 1 {
      }
      frame 2 {
      }
      frame 3 {
      }
      frame 4 {
      }
      frame Default {
      }
    }
    "Chassis_MoveMode" <- w370
    n184 = case shown="Default" w373 {
      tunnel: ["Gimbal_Prepare" "Gimbal_Stop" "Gimbal_RC_Mode" "Gimbal_Mouse_Mode" "Gimbal_Auto" "Gimbal_Standby" "Nothing"] -> w372
      frame 0 {
      }
      frame 1 {
      }
      frame 2 {
      }
      frame 3 {
      }
      frame 4 {
      }
      frame 5 {
      }
      frame Default {
      }
    }
    "Gimbal_MoveMode" <- w372
  }
  n185 = while {
    stop <- w416 stop-if-true
    w415 = FALSE
    # "Send instructions"
    n186 = local read "Serial port"() -> (w417:refnum<visa-resource-name>)
    n187 = event shown="[8] Timeout" {
      selector: _ -> [_ _ _ _ _ _ _ _ _]
      dyn-events: _ -> [_ _ _ _ _ _ _ _ _]
      timeout: u8 1 -> [_ _ _ _ _ _ _ _ _]
      tunnel: [w424 w430 w437 w454 w469 w486 w500 _ _] -> w418
      tunnel: w417 -> [w421 w429 w438 w444 w459 w485 w499 _ _]
      tunnel: [_ _ _ _ _ _ _ _ FALSE] -> w416
      event "Calibrate Gimbal": Value Change {
        n188 = event-data() -> ()  [unwired: 1 in, 1 out]
        n189 = VISA Write(VISA resource name=w421, write buffer="ª¯\u0001\u0001\u0005`") -> (return count=w423:u32, error out=w424:errorcluster)  [unwired: 1 in, 1 out]
        n190 = Greater Than 0?(x=w423) -> (x > 0?=w422:bool)
        n191 = case shown="True" w422 {
          tunnel: [FALSE TRUE] -> w420
          frame False {
          }
          frame True {
          }
        }
        "Calibrate Gimbal Susess" <- w420
      }
      event "Calibrate Gyro": Value Change {
        n192 = event-data() -> ()  [unwired: 1 in, 1 out]
        n193 = VISA Write(VISA resource name=w429, write buffer="ª¯\u0001\u0001\u0002]") -> (return count=w432:u32, error out=w430:errorcluster)  [unwired: 1 in, 1 out]
        n194 = Greater Than 0?(x=w432) -> (x > 0?=w431:bool)
        n195 = case shown="True" w431 {
          tunnel: [FALSE TRUE] -> w428
          frame False {
          }
          frame True {
          }
        }
        "Calibrate Gyro Susess" <- w428
      }
      event "Calibrate LittleGyro": Value Change {
        n196 = event-data() -> ()  [unwired: 1 in, 1 out]
        n197 = VISA Write(VISA resource name=w438, write buffer="ª¯\u0001\u0001\u0006a") -> (return count=w440:u32, error out=w437:errorcluster)  [unwired: 1 in, 1 out]
        n198 = Greater Than 0?(x=w440) -> (x > 0?=w441:bool)
        n199 = case shown="True" w441 {
          tunnel: [FALSE TRUE] -> w436
          frame False {
          }
          frame True {
          }
        }
        "Calibrate LittleGyro Susess" <- w436
      }
      event "Down Picth": Value Change {
        n200 = event-data() -> ()  [unwired: 1 in, 1 out]
        n201 = call "帧12打包.vi"("帧ID"=u8 16, "D 6"="P-S-D 2", "P1"="P-P-P 2", "I 5"="P-S-I 2", "P 4"="P-S-P 2", "D 3"="P-P-D 2", "I 2"="P-P-I 2") -> ("打包"=w445:string)
        n202 = VISA Write(VISA resource name=w444, write buffer=w445) -> (return count=w455:u32, error out=w454:errorcluster)  [unwired: 1 in, 1 out]
        n203 = Greater Than 0?(x=w455) -> (x > 0?=w456:bool)
        n204 = case shown="True" w456 {
          tunnel: [FALSE TRUE] -> w453
          frame False {
          }
          frame True {
          }
        }
        "Down Picth Susess" <- w453
      }
      event "Down Yaw": Value Change {
        n205 = event-data() -> ()  [unwired: 1 in, 1 out]
        n206 = call "帧12打包.vi"("帧ID"=u8 17, "D 6"="Y-S-D 2", "P1"="Y-P-P 2", "I 5"="Y-S-I 2", "P 4"="Y-S-P 2", "D 3"="Y-P-D 2", "I 2"="Y-P-I 2") -> ("打包"=w461:string)
        n207 = VISA Write(VISA resource name=w459, write buffer=w461) -> (return count=w471:u32, error out=w469:errorcluster)  [unwired: 1 in, 1 out]
        n208 = Greater Than 0?(x=w471) -> (x > 0?=w470:bool)
        n209 = case shown="False" w470 {
          tunnel: [FALSE TRUE] -> w468
          frame False {
          }
          frame True {
          }
        }
        "Down Yaw Susess" <- w468
      }
      event "Down Shoot": Value Change {
        n210 = event-data() -> ()  [unwired: 1 in, 1 out]
        n211 = call "帧16打包.vi"("帧ID"=u8 9, "8"="S-P-D", "1"="S-S-P", "7"="S-P-I", "2"="S-S-I", "6"="S-P-P", "5"="T-T-T-S", "4"="F-W-M-V", "3"="S-S-D") -> ("打包"=w483:string)  [unwired: 2 in]
        n212 = VISA Write(VISA resource name=w485, write buffer=w483) -> (return count=w488:u32, error out=w486:errorcluster)  [unwired: 1 in, 1 out]
        n213 = Greater Than 0?(x=w488) -> (x > 0?=w487:bool)
        n214 = case shown="False" w487 {
          tunnel: [FALSE TRUE] -> w474
          frame False {
          }
          frame True {
          }
        }
        "Down Shoot Susess" <- w474
      }
      event "Down Chassis": Value Change {
        n215 = event-data() -> ()  [unwired: 1 in, 1 out]
        n216 = call "帧12打包.vi"("帧ID"=u8 18, "D 6"="C-S-D", "P1"="R-S-P", "I 5"="C-S-I", "P 4"="C-S-P", "D 3"="R-S-D", "I 2"="R-S-I") -> ("打包"=w498:string)
        n217 = VISA Write(VISA resource name=w499, write buffer=w498) -> (return count=w501:u32, error out=w500:errorcluster)  [unwired: 1 in, 1 out]
        n218 = Greater Than 0?(x=w501) -> (x > 0?=w502:bool)
        n219 = case shown="False" w502 {
          tunnel: [FALSE TRUE] -> w497
          frame False {
          }
          frame True {
          }
        }
        "Down Chassis Susess" <- w497
      }
      event "Open": Key Down {
        n220 = event-data() -> ()  [unwired: 1 in, 1 out]
        "First?" <- TRUE
        "Init" <- 0
      }
      event Timeout {
        n221 = event-data() -> ()  [unwired: 1 in, 1 out]
      }
    }
    n222 = local write "Calibrate LittleGyro Susess"(w415) -> ()
    n223 = local write "Calibrate Gimbal Susess"(w415) -> ()
    n224 = local write "Down Picth Susess"(w415) -> ()
    n225 = local write "Down Yaw Susess"(w415) -> ()
    n226 = local write "Calibrate Gyro Susess"(w415) -> ()
    n227 = local write "Down Shoot Susess"(w415) -> ()
    n228 = local write "Down Chassis Susess"(w415) -> ()
    n229 = call <vilib>:"Simple Error Handler.vi"("error in (no error)"=w418) -> ()  [unwired: 1 in, 8 out]
  }
